vi "User Master.vi"(8 "error in (no error)":errorcluster) -> (0 "error out":errorcluster)   [LabVIEW 2017]
uses:
  Controls/Add User Icon.ctl
  Controls/User Viewer Icon.ctl
  <vilib>/addons/database/Connection.llb/DB Tools Open Connec (Path).vi
  Globle/Current date.vi
  <vilib>/addons/database/NI_Database_API.lvlib
panel:
  in  "Cancel Button - Archive":bool
  in  "Add User":bool
  out "element":string
  out "String 2":string
  out "Character Array":string[](array[string])
  out "Array":bool[](array[boolean])
  in  "Phone Number":i32 format="%10.0f"
  in  "User Name":string(combo)
  in  "Select Role":string(combo)
  out "Change Password indicator":T1
  in  "New Password":string
  in  "Old Password":string
  in  "Re-enter New Password":string
  in  "Change password":bool
  out "View User Indicator":T2
  in  "Password":string
  in  "Phone Number":string
  in  "E-mail":string
  in  "Username":string
  in  "Last Name":string
  in  "First Name":string
  out "Add user indicator":T1
  out "Table":string[][](table)
  in  "Password view":bool
  # "Add User"
  # "View User"
  # "Change Password"
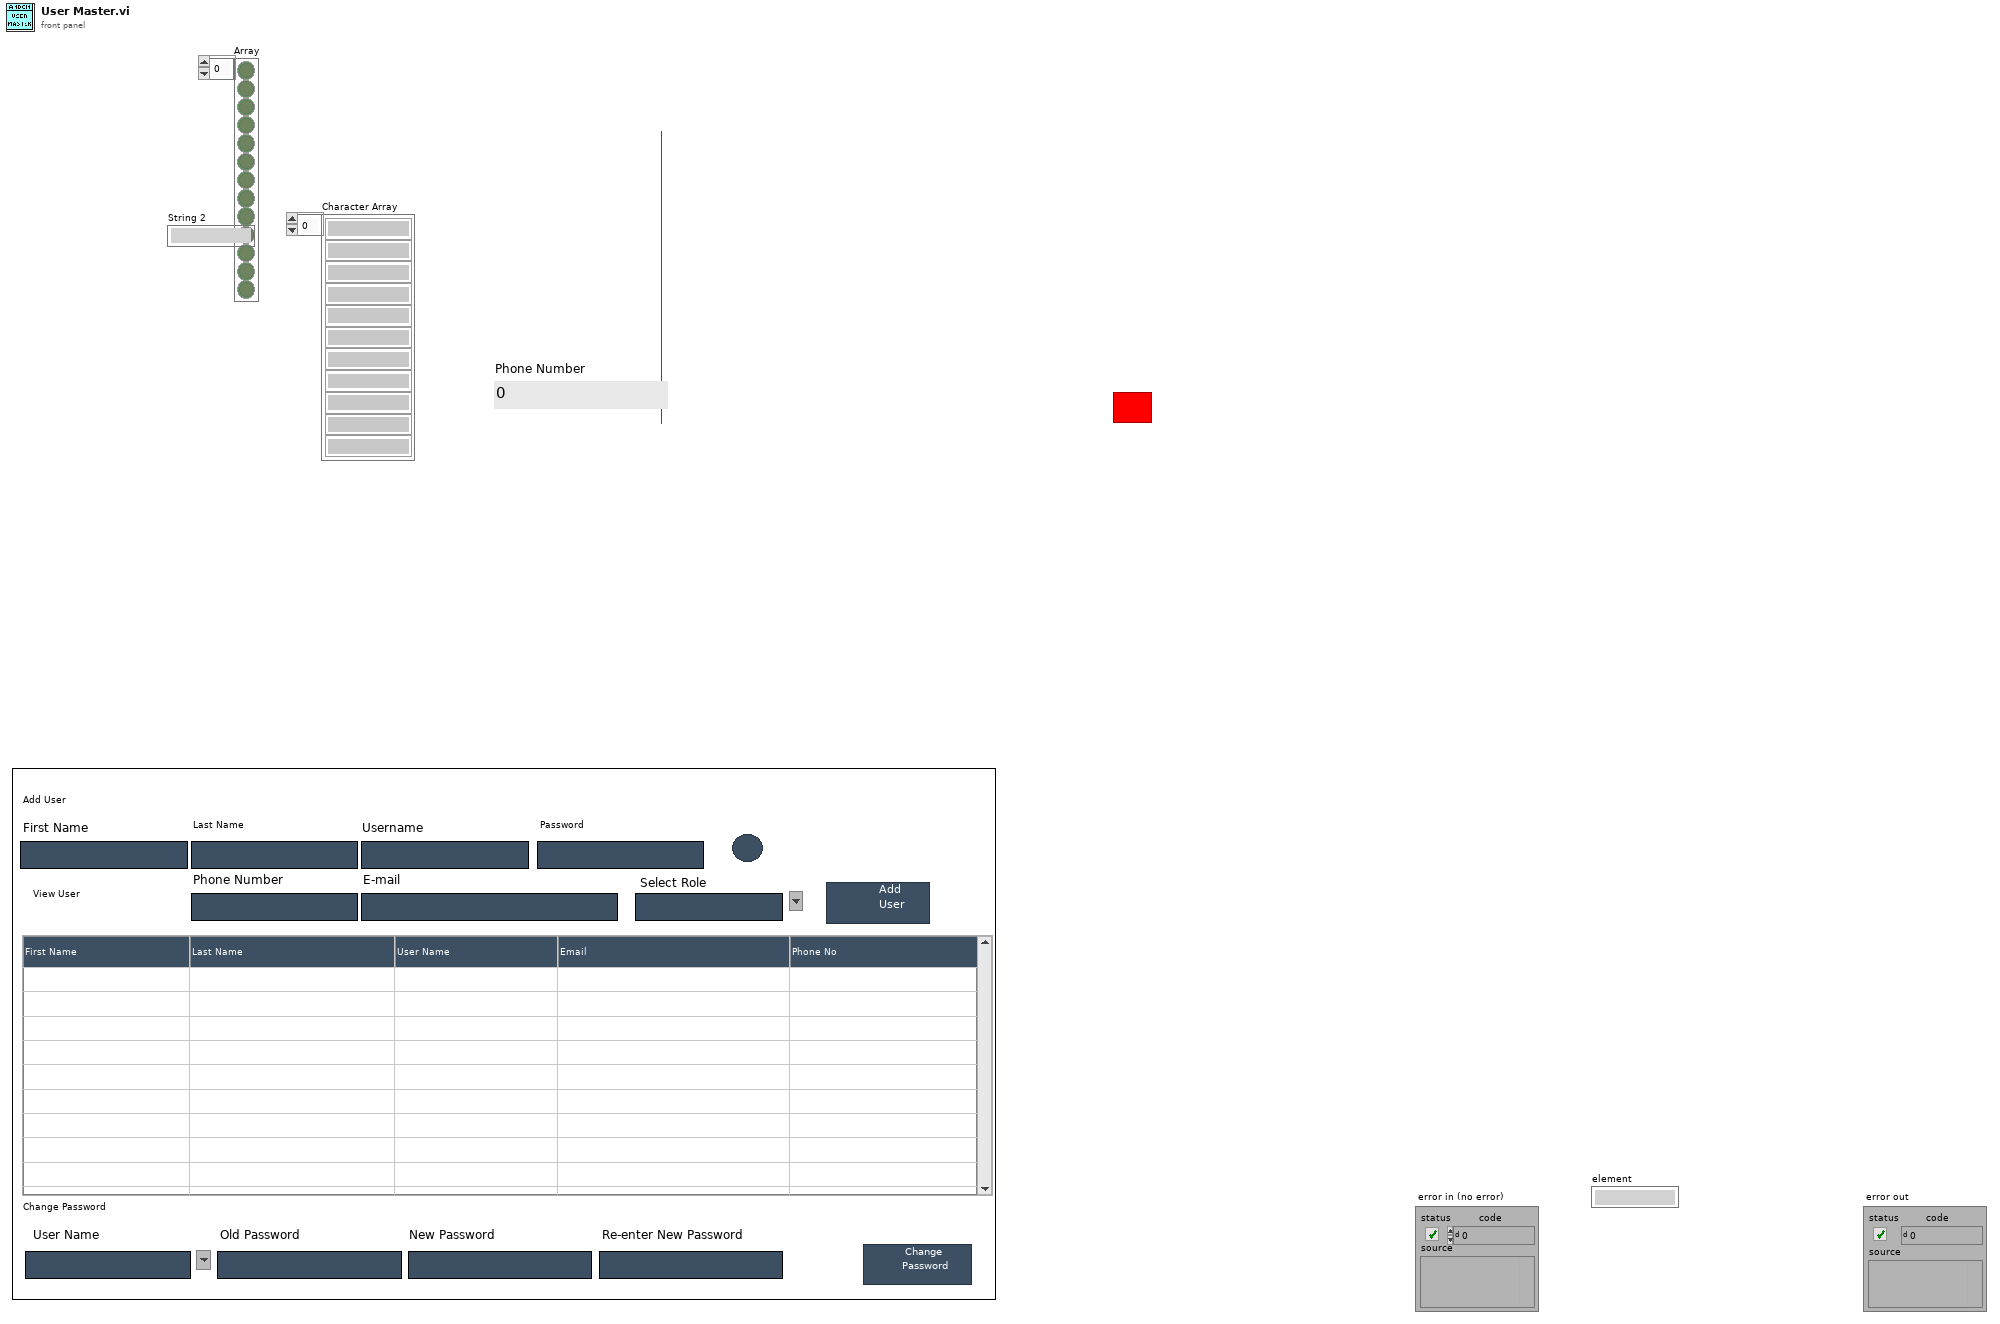
[diagram p1: front panel]
types:
  T1 = typedef "Add User Icon.ctl" = bool
  T2 = typedef "User Viewer Icon.ctl" = bool
  T3 = typedef "NI_Database_API.lvlib/Conn ObjectReference.ctl" = refnum<k1>
  T4 = cluster{"First Name":string, "Last Name":string, "Username":string, "string":string, "E-mail":string, "Phone Number":string, "Password":string, string}
  T5 = enum32{"invalid app kind", "Development System", "Run Time System", "Student Edition", "Embedded LabVIEW", "Evaluation", "Custom"}
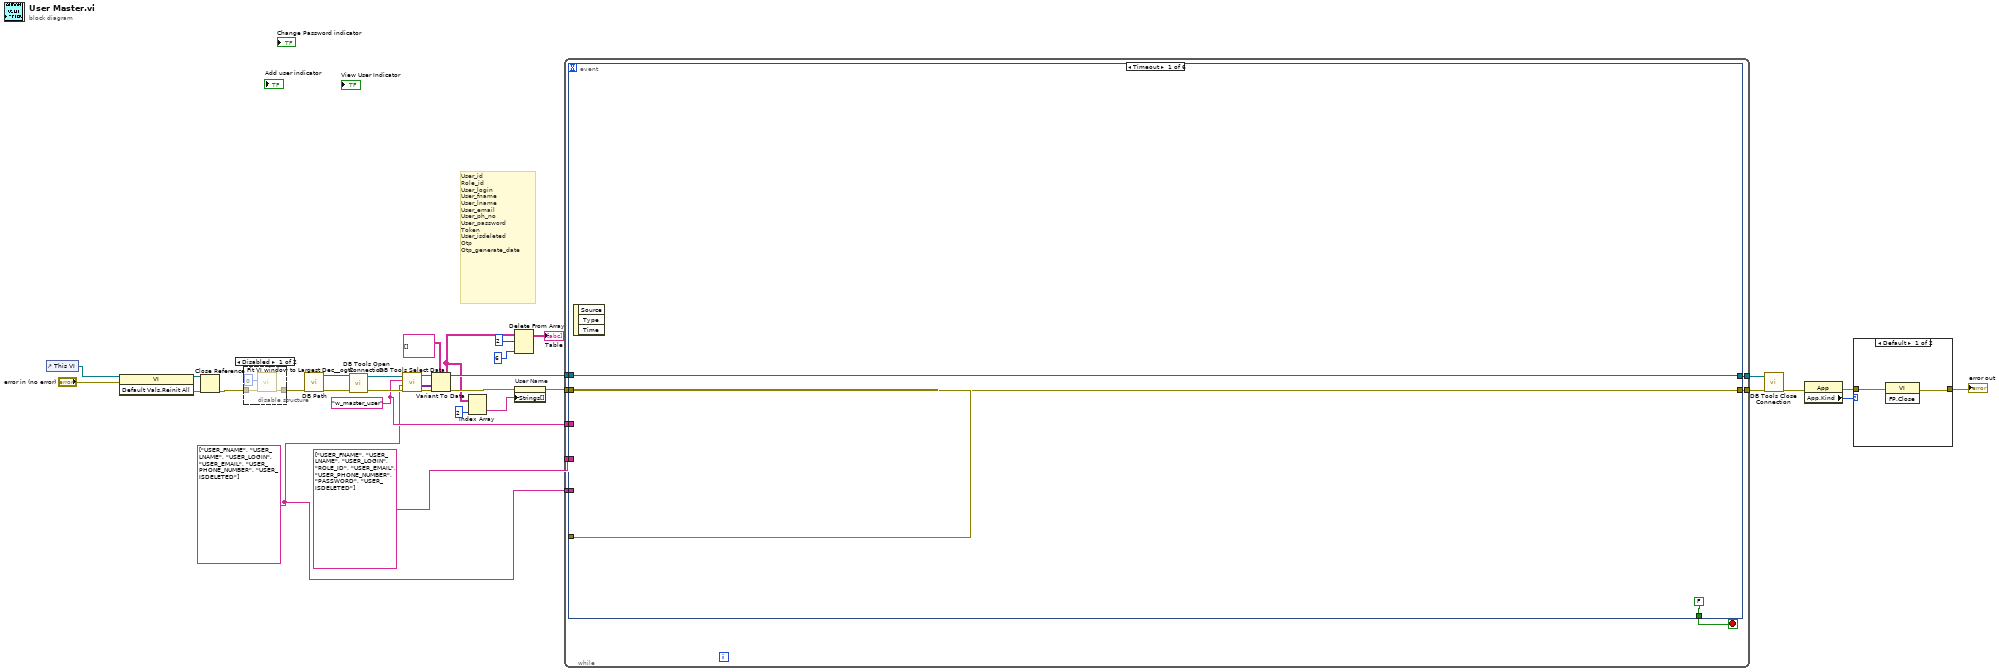
[diagram p0: block diagram]
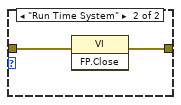
[diagram p3: hidden frame]
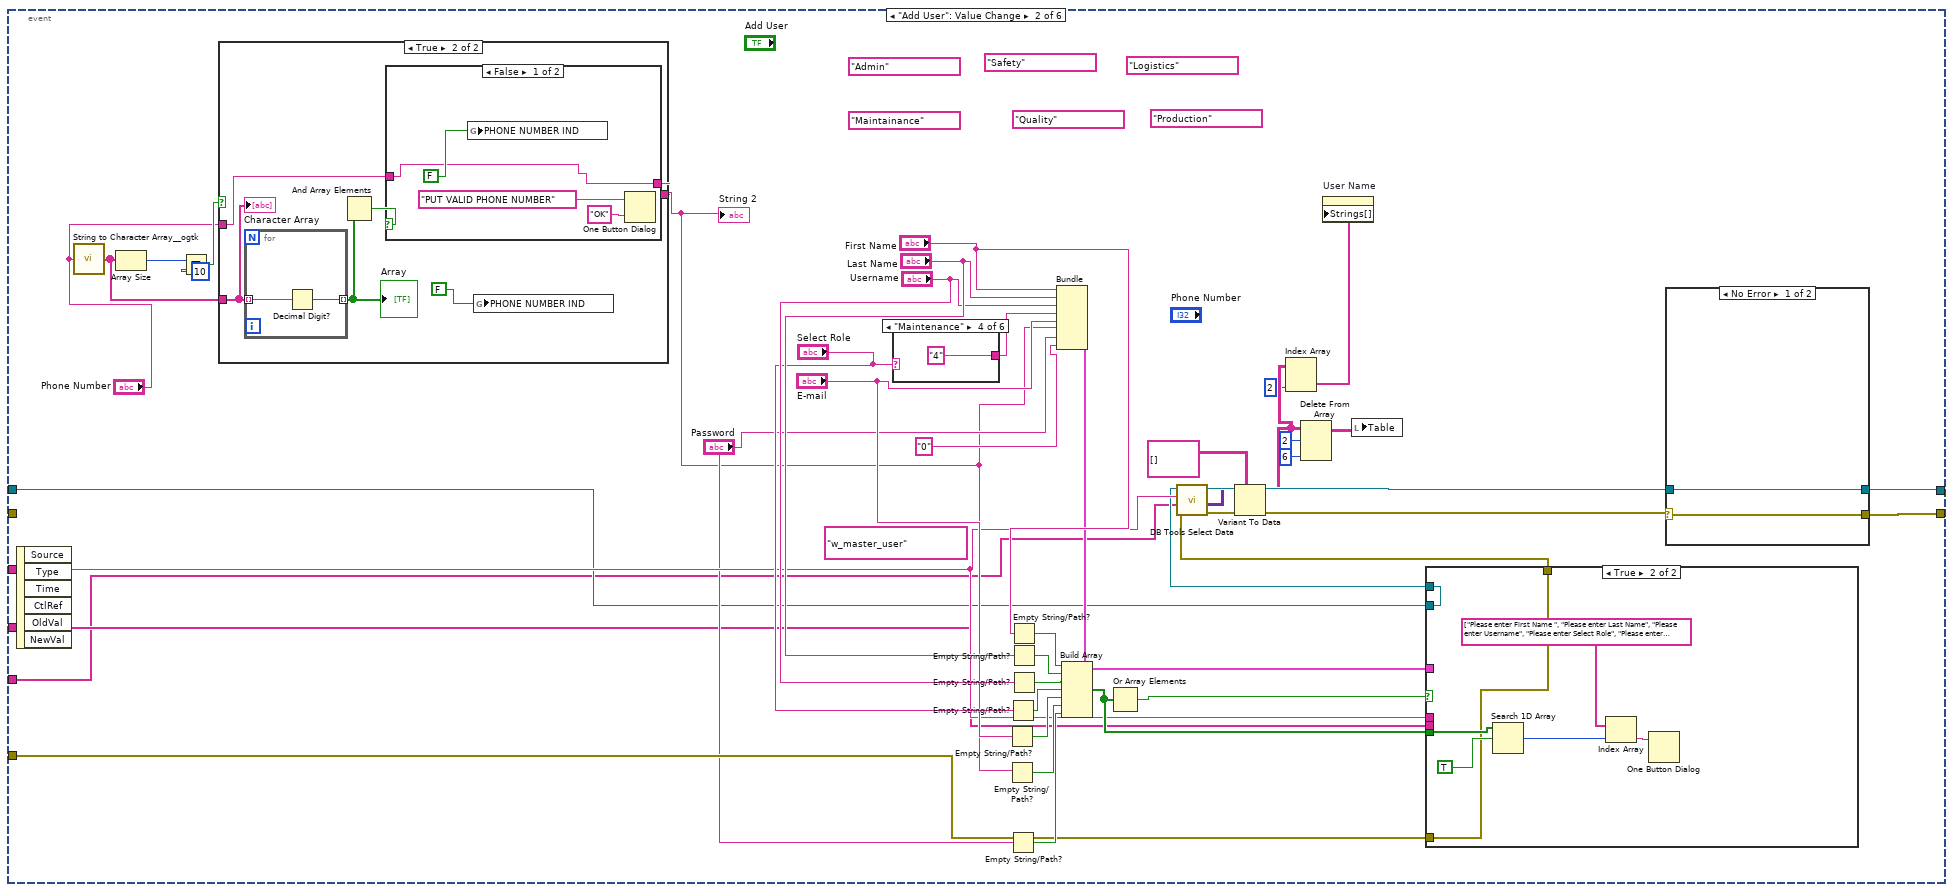
[diagram p4: hidden frame]
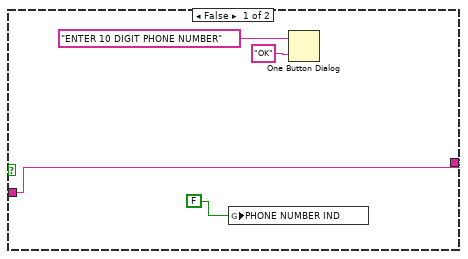
[diagram p5: hidden frame]
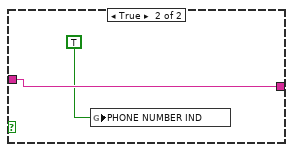
[diagram p6: hidden frame]
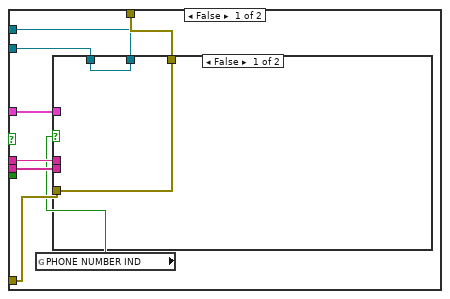
[diagram p7: hidden frame]
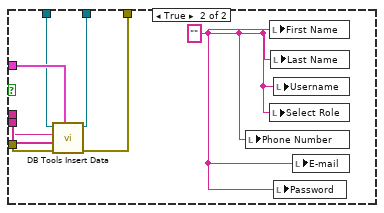
[diagram p8: hidden frame]
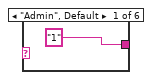
[diagram p10: hidden frame]
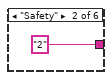
[diagram p11: hidden frame]
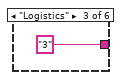
[diagram p12: hidden frame]
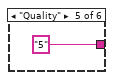
[diagram p13: hidden frame]
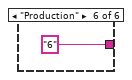
[diagram p14: hidden frame]
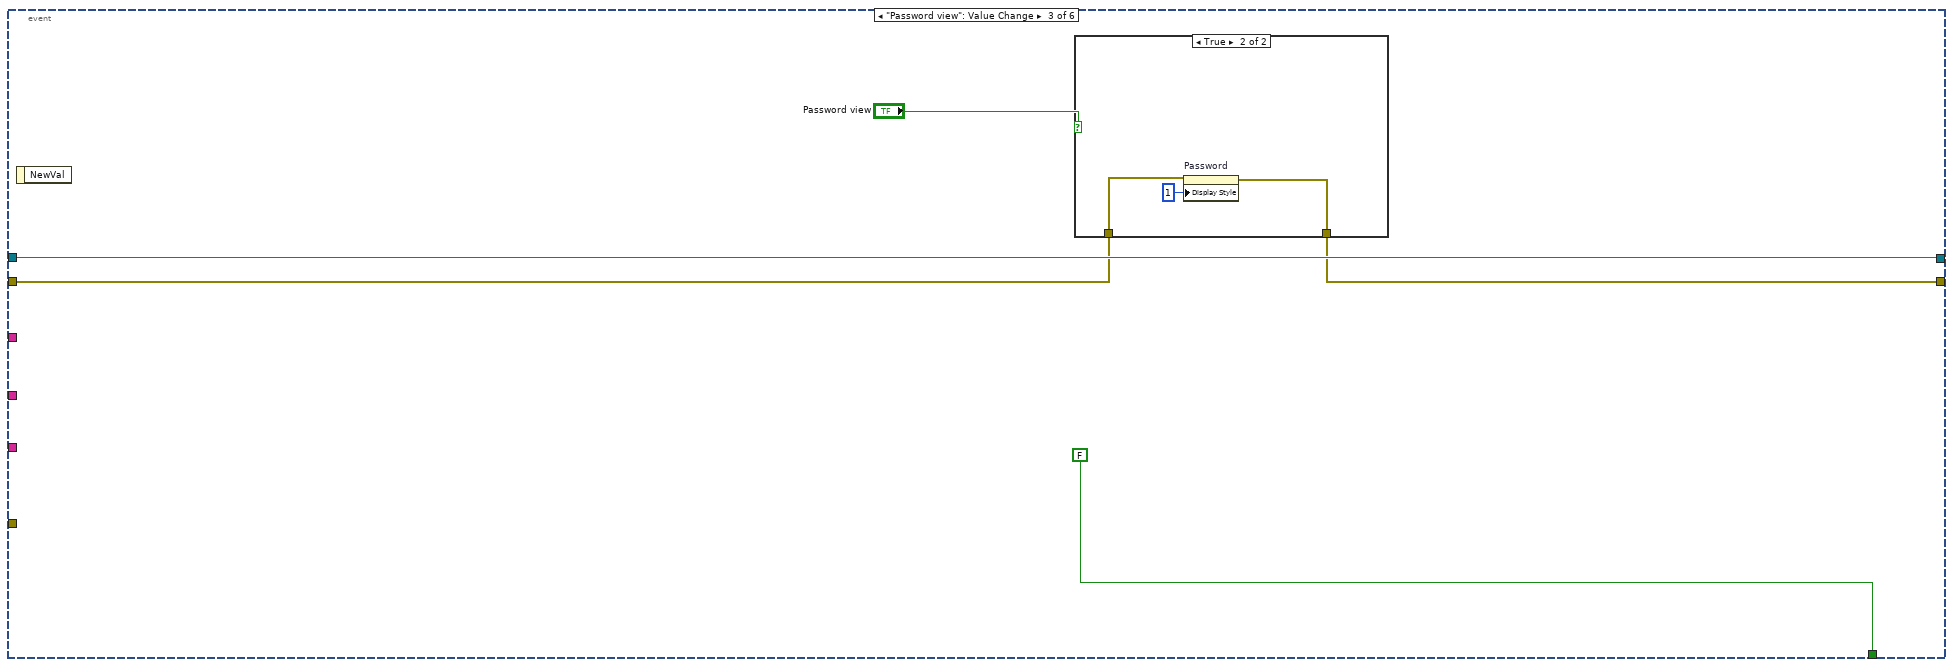
[diagram p15: hidden frame]
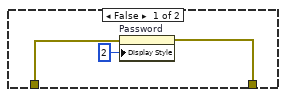
[diagram p16: hidden frame]
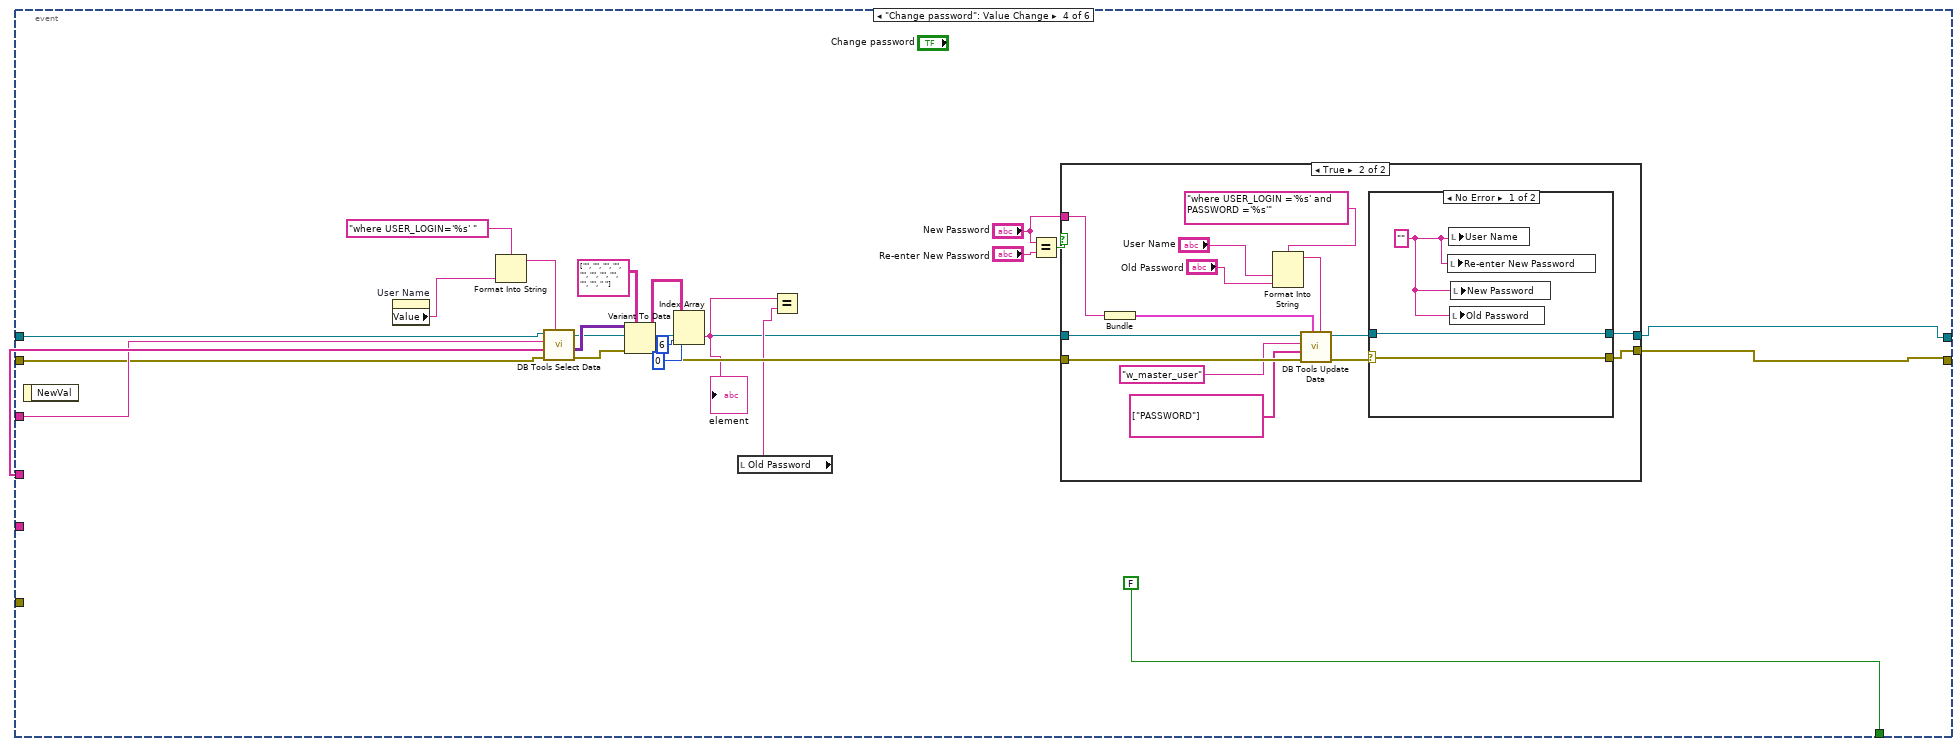
[diagram p17: hidden frame]
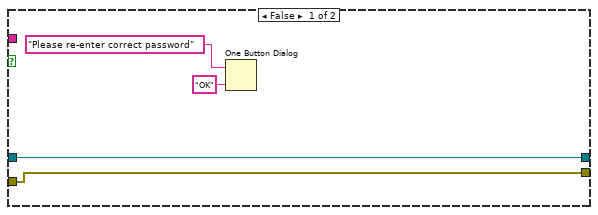
[diagram p18: hidden frame]
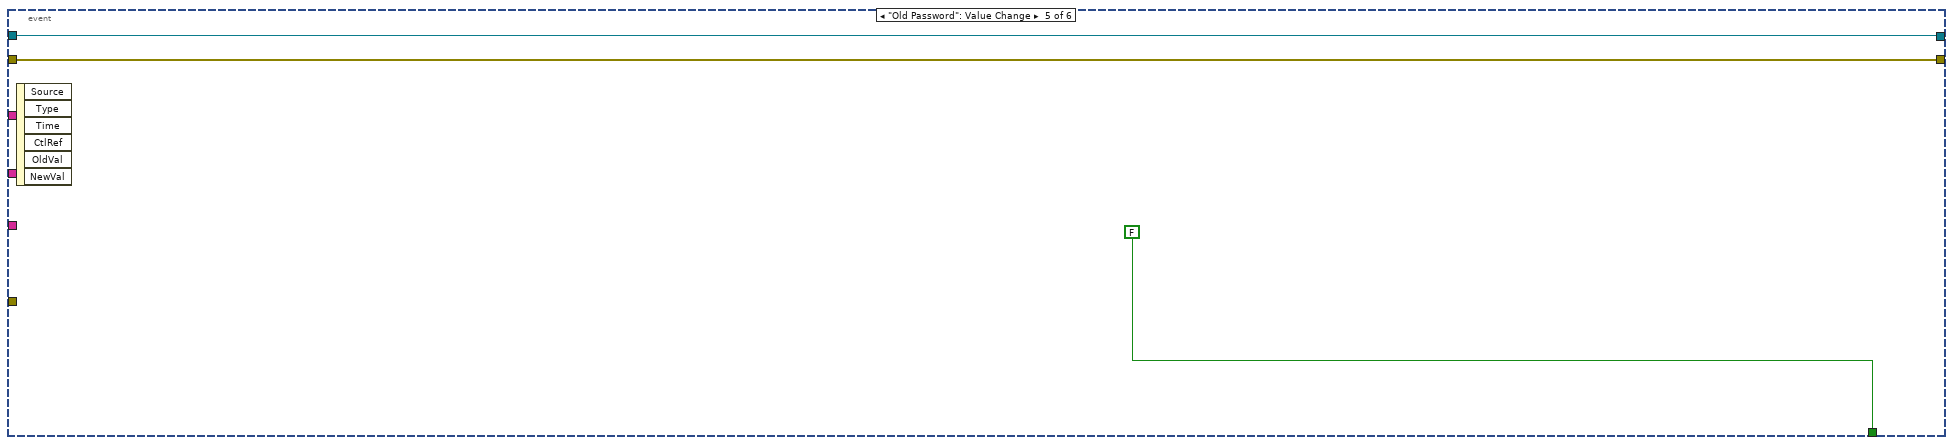
[diagram p20: hidden frame]
diagram:
  w1 = string[] ["USER_FNAME", "USER_LNAME", "USER_LOGIN", "USER_EMAIL", "USER_PHONE_NUMBER", "USER_ISDELETED"] ("columns")
  w6 = "w_master_user" ("table")
  # "User_id\nRole_id\nUser_login\nUser_fname\nUser_lname\nUser_email\nUser_ph_no\nUser_password\nToken\nUser_isdeleted\nOtp\nOtp_generate_date"
  n1 = control-ref of="This VI"() -> (w31:refnum<vi>)
  n2 = invoke class="VI" method="Default Vals.Reinit All"(reference=w31, error in="error in (no error)") -> (reference out=w28:refnum<vi>, error out=w29:errorcluster)  [unwired: 1 in, 1 out]
  n3 = Close Reference(reference=w28, error in (no error)=w29) -> (error out=w5:errorcluster)
  n4 = disable-structure shown="Disabled" {
    disable-tunnel: w5 -> [w34 w35]
    disable-tunnel: [w33 w35] -> w4
    frame Disabled {
      n5 = call <userlib>:"Fit VI window to Largest Dec__ogtk.vi"("error in (no error)"=w34, "border spacing (2 px)"=0) -> ("error out"=w33:errorcluster)  [unwired: 4 in, 1 out]
    }
    frame Enabled {
    }
  }
  n6 = call "DB Path.vi"("error in"=w4) -> ("error out"=w25:errorcluster, "DB Path"=w19:path)  [unwired: 9 in]
  n7 = call-poly <vilib>:"DB Tools Open Connection.vi"("error in (no error)"=w25, "connection information"=w19) -> ("error out"=w26:errorcluster, "connection reference"=w24:T3)  [unwired: 6 in]
  n8 = call <vilib>:"DB Tools Select Data.vi"("error in (no error)"=w26, "columns"=w1, "table"=w6, "connection reference"=w24) -> ("error out"=w18:errorcluster, "data"=w17:variant[][], "connection reference out"=w23:T3)  [unwired: 2 in]
  n9 = Variant To Data(error in=w18, type=string[][] [] ("Table"), Variant=w17) -> (data=w9:string[][], error out=w15:errorcluster)
  n10 = Index Array(array=w9, index (col)=2 ("disabled index (col)")) -> (element=w13:string[])  [unwired: 1 in]
  n11 = Delete From Array(array=w9, length=2, index (col)=6 ("disabled index (col)")) -> (array with subset deleted=→"Table":string[][])  [unwired: 1 in, 1 out]
  n12 = property on="User Name" class="CmbBox"(error in=w15, "Strings[]"=w13) -> (error out=w14:errorcluster)  [unwired: 1 in, 1 out]
  n13 = while {
    tunnel: w14 -> [w40]
    tunnel: [w42] -> w22
    tunnel: w23 -> [w37]
    tunnel: [w41] -> w20
    tunnel: string[] ["USER_FNAME", "USER_LNAME", "USER_LOGIN", "ROLE_ID", "USER_EMAIL", "USER_PHONE_NUMBER", "PASSWORD", "USER_ISDELETED"] ("columns") -> [w39]
    tunnel: w6 -> [w38]
    tunnel: w1 -> [w36]
    stop <- w43 stop-if-true
    n14 = event shown="[0] Timeout" {
      selector: _ -> [_ _ _ _ _ _]
      dyn-events: _ -> [_ _ _ _ _ _]
      timeout: _ -> [_ _ _ _ _ _]
      tunnel: w40 -> [w46 _ w146 w166 w201 w205]
      tunnel: [FALSE _ FALSE FALSE FALSE TRUE] -> w43
      tunnel: [w46 w90 w145 w158 w201 w205] -> w42
      tunnel: w37 -> [w45 w49 w148 w167 w202 w206]
      tunnel: [w45 w89 w148 w159 w202 w206] -> w41
      tunnel: w40 -> [_ w63 _ _ _ _]
      tunnel: w39 -> [_ w48 _ w176 _ _]
      tunnel: w38 -> [_ w62 _ w172 _ _]
      tunnel: w36 -> [_ w47 _ _ _ _]
      event Timeout {
        n15 = event-data() -> ()  [unwired: 1 in, 3 out]
      }
      event "Add User": Value Change {
        (unwired) "Production" ("Select Role")
        (unwired) "Quality" ("Select Role")
        (unwired) "Maintainance" ("Select Role")
        (unwired) "Logistics" ("Select Role")
        (unwired) "Safety" ("Select Role")
        (unwired) "Admin" ("Select Role")
        (unwired) "w_master_user" ("table")
        n16 = event-data() -> ()  [unwired: 1 in, 6 out]
        n17 = call <userlib>:"String to Character Array__ogtk.vi"("Input String"="Phone Number") -> ("Character Array"=w60:string[])
        n18 = Array Size(array=w60) -> (size(s)=w59:i32)
        n19 = Equal?(x=w59, y=10) -> (x = y?=w57:bool)
        n20 = case shown="True" w57 {
          tunnel: "Phone Number" -> [w91 w97]
          tunnel: w60 -> [_ w100]
          tunnel: [w91 w96] -> w54
          frame False {
            n21 = global write "Current date.vi" "PHONE NUMBER IND"(FALSE) -> ()
            n22 = One Button Dialog(message="ENTER 10 DIGIT PHONE NUMBER", button name ("OK")="OK") -> ()  [unwired: 1 out]
          }
          frame True {
            n23 = for {
              tunnel: w100 -> [w102] mode=indexing
              tunnel: [w101] -> w99 mode=indexing
              n24 = Decimal Digit?(1:w102) -> (0:w101:bool)
            }
            "Array" <- w99
            n25 = And Array Elements(Boolean array=w99) -> (logical AND=w98:bool)
            n26 = case shown="False" w98 {
              tunnel: w97 -> [w103 w108]
              tunnel: [w103 w108] -> w96
              frame False {
                n27 = global write "Current date.vi" "PHONE NUMBER IND"(FALSE) -> ()
                n28 = One Button Dialog(message="PUT VALID PHONE NUMBER", button name ("OK")="OK") -> ()  [unwired: 1 out]
              }
              frame True {
                n29 = global write "Current date.vi" "PHONE NUMBER IND"(TRUE ("PHONE NUMBER IND")) -> ()
              }
            }
            n30 = global write "Current date.vi" "PHONE NUMBER IND"(FALSE) -> ()
            "Character Array" <- w100
          }
        }
        "String 2" <- w54
        n31 = case shown="\"Maintenance\"" "Select Role" {
          tunnel: ["1" ("string") "2" "3" "4" "5" "6"] -> w80
          frame "Admin", Default {
          }
          frame "Safety" {
          }
          frame "Logistics" {
          }
          frame "Maintenance" {
          }
          frame "Quality" {
          }
          frame "Production" {
          }
        }
        n32 = Empty String/Path?(string/path="E-mail") -> (empty?=w78:bool)
        n33 = Empty String/Path?(string/path=w54) -> (empty?=w68:bool)
        n34 = Empty String/Path?(string/path="Select Role") -> (empty?=w77:bool)
        n35 = Empty String/Path?(string/path="Password") -> (empty?=w67:bool)
        n36 = Empty String/Path?(string/path="First Name") -> (empty?=w74:bool)
        n37 = Empty String/Path?(string/path="Last Name") -> (empty?=w75:bool)
        n38 = Empty String/Path?(string/path="Username") -> (empty?=w76:bool)
        n39 = Bundle("First Name"="First Name", "Last Name"="Last Name", "Username"="Username", "string"=w80, "E-mail"="E-mail", "Phone Number"=w54, "Password"="Password", "0") -> (w64:T4)  [unwired: 1 in]
        n40 = Build Array(w74, w75, w76, w77, w78, w68, w67) -> (w65:bool[])
        n41 = Or Array Elements(Boolean array=w65) -> (logical OR=w66:bool)
        n42 = case shown="True" w66 {
          tunnel: w65 -> [_ w129]
          tunnel: w64 -> [w116 _]
          tunnel: w63 -> [w115 w128]
          tunnel: w48 -> [w114 _]
          tunnel: w62 -> [w113 _]
          tunnel: [w112 w128] -> w61
          tunnel: [w111 w127] -> w50
          tunnel: w49 -> [w109 w127]
          frame False {
            n43 = global read "Current date.vi" "PHONE NUMBER IND"() -> (w110:bool)
            n44 = case shown="False" w110 {
              tunnel: w116 -> [_ w126]
              tunnel: w115 -> [w118 w125]
              tunnel: w114 -> [_ w124]
              tunnel: w113 -> [_ w123]
              tunnel: [w118 w122] -> w112
              tunnel: [w117 w121] -> w111
              tunnel: w109 -> [w117 w119]
              frame False {
              }
              frame True {
                w120 = ""
                n45 = call <vilib>:"DB Tools Insert Data.vi"("data"=w126, "error in (no error)"=w125, "columns"=w124, "table"=w123, "connection reference"=w119) -> ("error out"=w122:errorcluster, "connection reference out"=w121:T3)  [unwired: 5 in]
                n46 = local write "Phone Number"(w120) -> ()
                n47 = local write "First Name"(w120) -> ()
                n48 = local write "Select Role"(w120) -> ()
                n49 = local write "Last Name"(w120) -> ()
                n50 = local write "Username"(w120) -> ()
                n51 = local write "Password"(w120) -> ()
                n52 = local write "E-mail"(w120) -> ()
              }
            }
          }
          frame True {
            n53 = Search 1D Array(1D array=w129, element=TRUE) -> (index of element=w132:i32)  [unwired: 1 in]
            n54 = Index Array(array=string[] ["Please enter First Name ", "Please enter Last Name", "Please enter Username", "Please enter Select Role", "Please enter E-mail", "Please enter PHONE NUMBER ", "Password"], index=w132) -> (element=w130:string)
            n55 = One Button Dialog(message=w130) -> ()  [unwired: 1 in, 1 out]
          }
        }
        n56 = call <vilib>:"DB Tools Select Data.vi"("error in (no error)"=w61, "columns"=w47, "table"=w62, "connection reference"=w50) -> ("error out"=w86:errorcluster, "data"=w87:variant[][], "connection reference out"=w88:T3)  [unwired: 2 in]
        n57 = Variant To Data(error in=w86, type=string[][] [] ("Table"), Variant=w87) -> (data=w53:string[][], error out=w85:errorcluster)
        n58 = Index Array(array=w53, index (col)=2 ("disabled index (col)")) -> (element=w51:string[])  [unwired: 1 in]
        n59 = Delete From Array(array=w53, length=2, index (col)=6 ("disabled index (col)")) -> (array with subset deleted=w81:string[][])  [unwired: 1 in, 1 out]
        n60 = property on="User Name" class="CmbBox"("Strings[]"=w51) -> ()  [unwired: 2 in, 2 out]
        n61 = local write "Table"(w81) -> ()
        n62 = case shown="No Error" w85 {
          selector: w85 -> [w135 w137]
          tunnel: [w135 w137] -> w90
          tunnel: w88 -> [w134 w136]
          tunnel: [w134 w136] -> w89
          frame No Error {
          }
          frame Error {
          }
        }
      }
      event "Password view": Value Change {
        n63 = event-data() -> ()  [unwired: 1 in, 1 out]
        n64 = case shown="True" "Password view" {
          tunnel: w146 -> [w151 w154]
          tunnel: [w150 w153] -> w145
          frame False {
            n65 = property on="Password" class="Str"(error in=w151, "Display Style"=u32 2) -> (error out=w150:errorcluster)  [unwired: 1 in, 1 out]
          }
          frame True {
            n66 = property on="Password" class="Str"(error in=w154, "Display Style"=u32 1) -> (error out=w153:errorcluster)  [unwired: 1 in, 1 out]
          }
        }
      }
      event "Change password": Value Change {
        n67 = event-data() -> ()  [unwired: 1 in, 1 out]
        n68 = property on="User Name" class="CmbBox"() -> ("Value"=w174:string)  [unwired: 2 in, 2 out]
        n69 = Format Into String(format string="where USER_LOGIN='%s' ", w174) -> (resulting string=w173:string)  [unwired: 2 in, 1 out]
        n70 = call <vilib>:"DB Tools Select Data.vi"("condition"=w173, "error in (no error)"=w166, "columns"=w176, "table"=w172, "connection reference"=w167) -> ("error out"=w164:errorcluster, "data"=w171:variant[][], "connection reference out"=w160:T3)  [unwired: 1 in]
        n71 = Variant To Data(error in=w164, type=string[][] [["", "", "", "", "", "", "", "", "", "", " "]] ("Table"), Variant=w171) -> (data=w169:string[][], error out=w163:errorcluster)
        n72 = Index Array(array=w169, index (row)=0 ("disabled index (row)"), index (col)=6 ("disabled index (col)")) -> (element=w162:string)
        "element" <- w162
        n73 = local read "Old Password"() -> (w161:string)
        n74 = Equal?(x=w162, y=w161) -> ()  [unwired: 1 out]
        n75 = Equal?(x="New Password", y="Re-enter New Password") -> (x = y?=w155:bool)
        n76 = case shown="True" w155 {
          tunnel: w163 -> [w178 w195]
          tunnel: [w181 w182] -> w159
          tunnel: w160 -> [w181 w194]
          tunnel: "New Password" -> [_ w191]
          tunnel: [w178 w183] -> w158
          frame False {
            n77 = One Button Dialog(message="Please re-enter correct password", button name ("OK")="OK") -> ()  [unwired: 1 out]
          }
          frame True {
            n78 = Bundle("New Password"=w191) -> (w190:cluster{"New Password":string})  [unwired: 1 in]
            n79 = Format Into String(format string="where USER_LOGIN ='%s' and PASSWORD ='%s'", "User Name", "Old Password") -> (resulting string=w186:string)  [unwired: 2 in, 1 out]
            n80 = call <vilib>:"DB Tools Update Data.vi"("condition"=w186, "data"=w190, "error in (no error)"=w195, "columns"=string[] ["PASSWORD"], "table"="w_master_user", "connection reference"=w194) -> ("error out"=w185:errorcluster, "connection reference out"=w184:T3)  [unwired: 4 in]
            n81 = case shown="No Error" w185 {
              selector: w185 -> [w197 w199]
              tunnel: w184 -> [w198 w200]
              tunnel: [w198 w200] -> w182
              tunnel: [w197 w199] -> w183
              frame No Error {
                w196 = ""
                n82 = local write "Re-enter New Password"(w196) -> ()
                n83 = local write "User Name"(w196) -> ()
                n84 = local write "Old Password"(w196) -> ()
                n85 = local write "New Password"(w196) -> ()
              }
              frame Error {
              }
            }
          }
        }
      }
      event "Old Password": Value Change {
        n86 = event-data() -> ()  [unwired: 1 in, 6 out]
      }
      event "Cancel Button - Archive": Value Change {
        n87 = event-data() -> ()  [unwired: 1 in, 6 out]
      }
    }
  }
  n88 = call <vilib>:"DB Tools Close Connection.vi"("error in (no error)"=w22, "connection reference"=w20) -> ("error out"=w21:errorcluster)  [unwired: 5 in]
  n89 = property class="App"(error in=w21) -> (error out=w2:errorcluster, "App.Kind"=w3:T5)  [unwired: 1 in, 1 out]
  n90 = case shown="Default" w3 {
    tunnel: w2 -> [w208 w210]
    tunnel: [w207 w209] -> w27
    frame Default {
      n91 = invoke class="VI" method="FP.Close"(error in=w208) -> (error out=w207:errorcluster)  [unwired: 2 in, 2 out]
    }
    frame "Run Time System" {
      n92 = invoke class="VI" method="FP.Close"(error in=w210) -> (error out=w209:errorcluster)  [unwired: 2 in, 2 out]
    }
  }
  "error out" <- w27
